vi "Test.vi"   [LabVIEW 2014]
doc: "This VI is called when test mode begins, and will automatically be terminated when it ends. You can add manual or automatic tests and invoke them from the dashboard."
uses:
  <vilib>/Rock Robotics/WPI/RobotDrive/WPI_RobotDriveGetSetRefNum.vi
  <vilib>/addons/control/pid/pid.llb/PID (DBL).vi
  <vilib>/Rock Robotics/WPI/RobotDrive/WPI_RobotDriveMecanumDrive_Cartesian.vi
  <vilib>/addons/control/pid/NI_PID_pid.lvlib
types:
  T1 = typedef "WPI_GyroDevRef.ctl" = cluster{"DevStatus":errorcluster, "Analog Module":T2, "Analog Channel":T3, "Offset":dbl, "Gain (VoltsPerDegree/Second)":dbl}
  T2 = typedef "FPGA_TypedefAnalogModule.ctl" = enum16{"Controller 1"}
  T3 = typedef "FPGA_AIChannel.ctl" = enum8{"AI 0", "AI 1", "AI 2", "AI 3", "AI MXP 0", "AI MXP 1", "AI MXP 2", "AI MXP 3", "Invalid"}
  T4 = typedef "WPI_RobotDriveDevRef.ctl" = cluster{"DevStatus":errorcluster, "Motors[]":T5[], "Square Inputs":bool, "Max Output":dbl}
  T5 = typedef "WPI_MotorControlDeviceRef.ctl" = cluster{"DeviceStatus":errorcluster, "Type":T6, "PWM":cluster{"Controller":T7, "PWM Channel":T8, "DeadBand":T9}, "CAN":cluster{"Device Number":u8, "Control Mode":T10, "Semaphore":T11, "Max Vout":dbl, "TalonSRX Control Mode":T12}, "Invert":bool, "TransformRef":T13, "InvTransformRef":T13}
  T6 = typedef "WPI_MotorControlType.ctl" = enum16{"PWM", "CAN", "CANTalonSRX"}
  T7 = typedef "FPGA_TypedefDigitalModule.ctl" = enum16{"Controller 1"}
  T8 = typedef "FPGA_DIOPWMChannel.ctl" = enum8{"PWM 0", "PWM 1", "PWM 2", "PWM 3", "PWM 4", "PWM 5", "PWM 6", "PWM 7", "PWM 8", "PWM 9", "PWM MXP 0", "PWM MXP 1", "PWM MXP 2", "PWM MXP 3", "PWM MXP 4", "PWM MXP 5", "PWM MXP 6", "PWM MXP 7", "PWM MXP 8", "PWM MXP 9", "Invalid"}
  T9 = typedef "WPI_PWMDeadband.ctl" = cluster{"Name":string, "maxPositivePwm":i32, "minPositivePwm":i32, "centerPwm":i32, "maxNegativePwm":i32, "minNegativePwm":i32, "angularRange":u16}
  T10 = typedef "WPI_CANJaguar_ControlMode.ctl" = enum8{"Percent VBus", "Current", "Speed", "Position", "Voltage"}
  T11 = typedef "Semaphore RefNum" = refnum<k1>
  T12 = typedef "WPI_CANTalonSRX_APIControlMode.ctl" = enum8{"Percent VBus", "Speed", "Position", "Slave", "Unchanged / Invalid"}
  T13 = typedef "WPI_PWMTransform_ConPane.ctl" = refnum<vi>
  T14 = cluster{"proportional gain (Kc)":dbl, "integral time (Ti, min)":dbl, "derivative time (Td, min)":dbl}
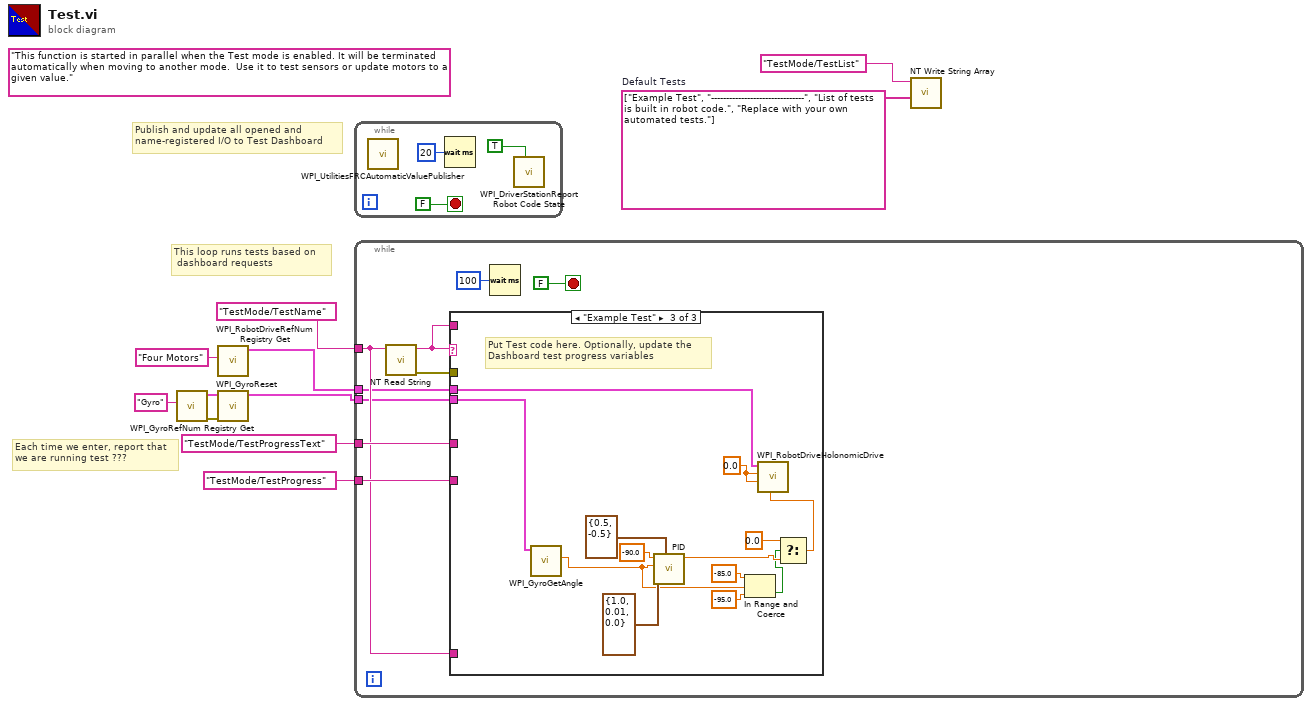
[diagram p0: block diagram]
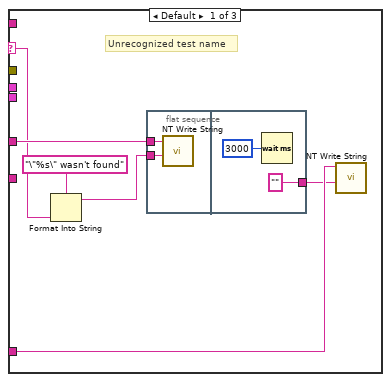
[diagram p2: hidden frame]
diagram:
  w8 = string[] ["Example Test", "-------------------------------", "List of tests is built in robot code.", "Replace with your own automated tests."]  # Default Tests
  (unwired) "This function is started in parallel when the Test mode is enabled. It will be terminated automatically when moving to another mode.  Use it to test sensors or update motors to a given value."
  # "This loop runs tests based on \n dashboard requests"
  # "Publish and update all opened and\nname-registered I/O to Test Dashboard"
  # "Each time we enter, report that\nwe are running test ???"
  n1 = call <vilib>:"WPI_GyroRefNum Registry Get.vi"("refnum name"="Gyro") -> ("error out"=w6:errorcluster, "GyroDevRef"=w5:T1)  [unwired: 9 in]
  n2 = call <vilib>:"WPI_RobotDriveRefNum Registry Get.vi"("refnum name"="Four Motors") -> ("RobotDriveDevRef"=w2:T4)  [unwired: 9 in, 1 out]
  n3 = call <vilib>:"WPI_GyroReset.vi"("error in (no error)"=w6, "GyroDevRef"=w5) -> ("GyroDevRef"=w1:T1)  [unwired: 8 in, 1 out]
  n4 = while {
    stop <- FALSE stop-if-true
    n5 = call <vilib>:"WPI_UtilitiesFRCAutomaticValuePublisher.vi"() -> ()  [unwired: 12 in]
    n6 = Wait (ms)(milliseconds to wait=u32 20) -> ()  [unwired: 1 out]
    n7 = call <vilib>:"WPI_DriverStationReport Robot Code State.vi"("Test"=TRUE ("Autonomous")) -> ()  [unwired: 10 in, 1 out]
  }
  n8 = while {
    tunnel: "TestMode/TestName" ("Name") -> [w18]
    tunnel: "TestMode/TestProgressText" ("Name") -> [w21]
    tunnel: "TestMode/TestProgress" ("Name") -> [w20]
    tunnel: w2 -> [w16]
    tunnel: w1 -> [w15]
    stop <- FALSE stop-if-true
    n9 = call <vilib>:"NT Read String.vi"("Name"=w18) -> ("error out"=w17:errorcluster, "String"=w19:string)  [unwired: 9 in]
    n10 = case shown="\"Example Test\"" w19 {
      selector: w19 -> [w28 _ _]
      tunnel: w18 -> [w25 _ _]
      tunnel: w21 -> [w29 _ _]
      tunnel: w20 -> [_ _ _]
      tunnel: w19 -> [_ _ _]
      tunnel: w17 -> [_ _ _]
      tunnel: w16 -> [_ _ w37]
      tunnel: w15 -> [_ _ w36]
      frame Default {
        # "Unrecognized test name"
        n11 = Format Into String(format string="\"%s\" wasn't found" ("Name"), w28) -> (resulting string=w27:string)  [unwired: 2 in, 1 out]
        n12 = flat-sequence {
          tunnel: w29 -> [w30]
          tunnel: w27 -> [w31]
          tunnel: ["" ("Name")] -> w24
          frame #0 {
            n13 = call <vilib>:"NT Write String.vi"("String"=w31, "Name"=w30) -> ()  [unwired: 9 in, 1 out]
          }
          frame #1 {
            n14 = Wait (ms)(milliseconds to wait=u32 3000) -> ()  [unwired: 1 out]
          }
        }
        n15 = call <vilib>:"NT Write String.vi"("String"=w24, "Name"=w25) -> ()  [unwired: 9 in, 1 out]
      }
      frame "" {
        # "No test to run"
      }
      frame "Example Test" {
        w40 = 0.0 ("X")
        # "Put Test code here. Optionally, update the\nDashboard test progress variables"
        n16 = call <vilib>:"WPI_GyroGetAngle.vi"("GyroDevRef"=w36) -> ("Angle"=w34:dbl)  [unwired: 7 in, 3 out]
        n17 = call-poly <vilib>:"PID.vi"("output range"=cluster{"output high":dbl, "output low":dbl} {"output high"=0.5, "output low"=-0.5}, "PID gains"=T14 {"proportional gain (Kc)"=1.0, "integral time (Ti, min)"=0.01, "derivative time (Td, min)"=0.0}, "process variable"=w34, "setpoint"=-90.0) -> ("output"=w44:dbl)  [unwired: 6 in, 1 out]
        n18 = In Range and Coerce(upper limit=-85.0, x=w34, lower limit=-95.0) -> (In Range?=w43:bool)  [unwired: 1 out]
        n19 = Select(t=0.0, s=w43, f=w44) -> (s? t:f=w45:dbl)
        n20 = call-poly <vilib>:"WPI_RobotDriveHolonomicDrive.vi"("Rotation"=w45, "y"=w40, "X"=w40, "RobotDriveDevRef"=w37) -> ()  [unwired: 5 in, 3 out]
      }
    }
    n21 = Wait (ms)(milliseconds to wait=u32 100) -> ()  [unwired: 1 out]
  }
  n22 = call <vilib>:"NT Write String Array.vi"("String Array"=w8, "Name"="TestMode/TestList") -> ()  [unwired: 9 in, 1 out]
